vi "prepDO_focusalign.vi"(2 "rate":dbl=30000.0 format="%#_13g", 3 "data":digitalwaveform[](array[waveform]), 4 "bufferAO":i32) -> (0 "error out":errorcluster, 1 "task out":refnum<k21>)   [LabVIEW 2015]
uses:
  <vilib>/DAQmx/write.llb/DAQmx Write (Digital 1D Wfm NChan NSamp).vi
  <vilib>/DAQmx/create/channels.llb/DAQmx Create Channel (DO-Digital Output).vi
  <vilib>/DAQmx/configure/timing.llb/DAQmx Timing (Sample Clock).vi
  <vilib>/Waveform/DWDTOps.llb/DWDT Uncompress Digital.vi
  <vilib>/DAQmx/miscellaneous.llb/DAQmx Fill In Error Info.vi
panel:
  in  "error in":errorcluster
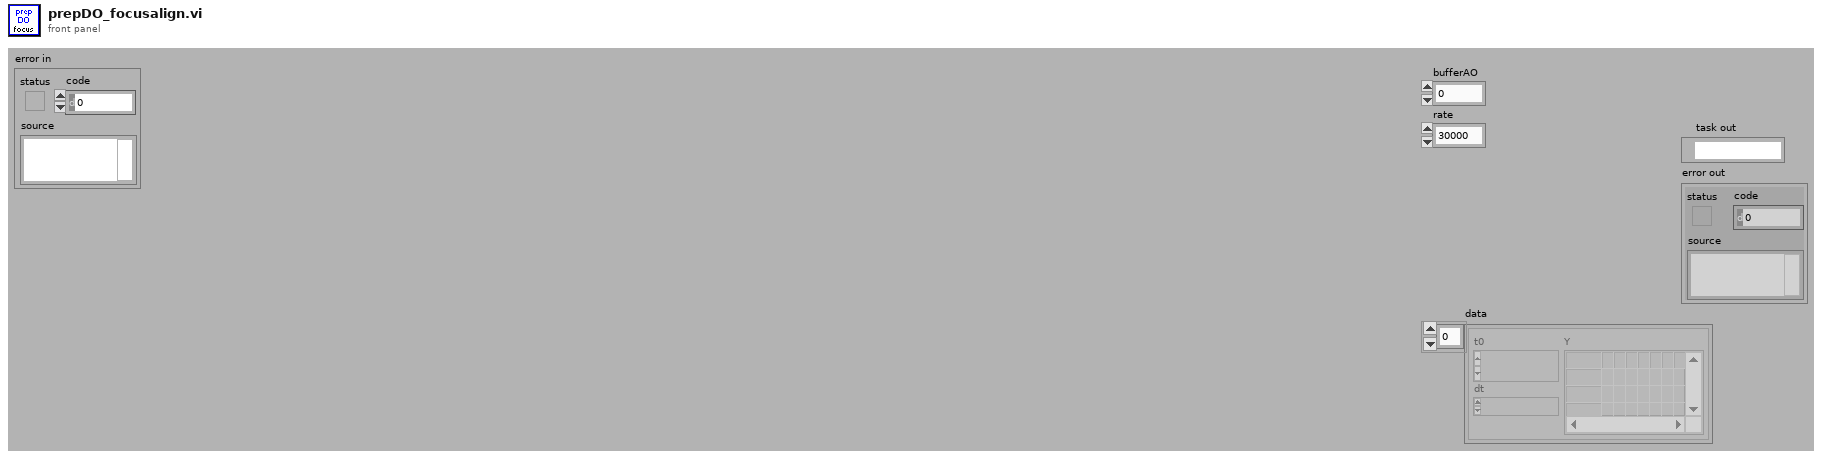
[diagram p1: front panel]
types:
  T1 = cluster{"StageS":i32, "StageL":i32, "currmeas data dir":path, "image OD":u16, "contour OD":u16, "point OD":u16, "AOlines":tag[], "AIlines":tag[], "CI lines":tag[], "DO lines":tag[], "AO names":string[], "CI names":string[], "AI names":string[], "DO names":string[], "CIextensions":string[], "AIextensions":string[], "Voltage to Ygalvo":i32, "Voltage to Xgalvo":i32, "Voltage to patch":i32, "640 shutter":i32, "2P shutter":i32, "LT timestamp":u32, "Vp":i32, "Ip":i32, "camera trigger":i32, "master data dir":path, "voltage to Zpos":i32, "Vto2P":i32, "640 AO":i32, "488 AO":i32, "532 AO":i32, "640TTL":u32, "488TTL":u32, "532TTL":u32, "Device 1 sampleclock out":tag, "Device 1 Starttrigger out":tag, "Device 2 sampleclock in":tag, "Device 2 StartTrigger in ":tag, "2PODTTL":u32, "488 shutter":u32, "LCVR red":u32, "LCVR blue":u32}
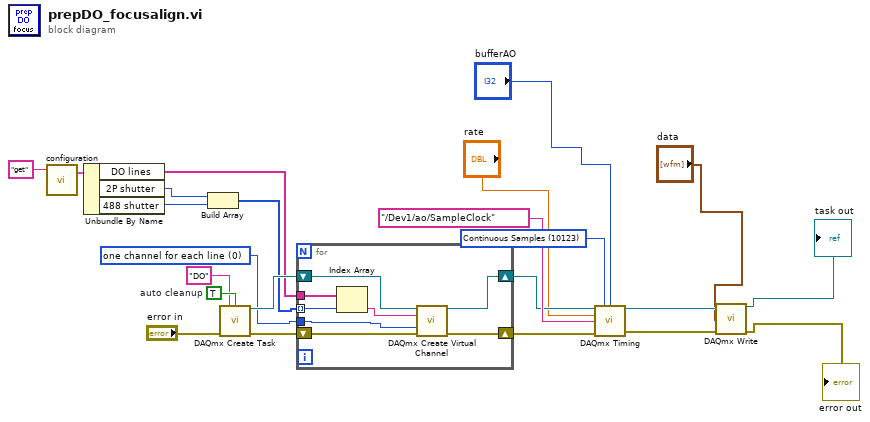
[diagram p0: block diagram]
diagram:
  w7 = 10123 items=["Finite Samples"=10178, "Continuous Samples"=10123, "Hardware Timed Single Point"=12522] ("sample mode")
  w13 = 0 items=["one channel for each line", "one channel for all lines"] ("line grouping")
  w22 = TRUE  # auto cleanup
  n1 = call "configuration.vi"("command"="get") -> ("config out"=w15:T1)  [unwired: 2 in, 1 out]
  n2 = Unbundle By Name(w15) -> ("DO lines"=w14:tag[], "2P shutter"=w5:i32, "488 shutter"=w4:u32)
  n3 = Build Array(w5, w4) -> (w3:u32[])
  n4 = call <vilib>:"DAQmx Create Task.vi"("new task name"="DO", "auto cleanup"=w22, "error in"="error in") -> ("task out"=w23:refnum<k21>, "error out"=w21:errorcluster)  [unwired: 11 in]
  n5 = for {
    shift-right: [w26] -> w17
    shift-left: w21 -> [w30]
    tunnel: w3 -> [w29] mode=indexing
    shift-right: [w27] -> w18
    shift-left: w23 -> [w31]
    tunnel: w14 -> [w25]
    tunnel: w13 -> [w24]
    n6 = Index Array(array=w25, index=w29) -> (element=w28:tag)
    n7 = call-poly <vilib>:"DAQmx Create Virtual Channel.vi"("task in"=w31, "lines"=w28, "line grouping"=w24, "error in"=w30) -> ("task out"=w27:refnum<k21>, "error out"=w26:errorcluster)  [unwired: 10 in]
  }
  n8 = call-poly <vilib>:"DAQmx Timing.vi"("task/channels in"=w18, "sample mode"=w7, "samples per channel"="bufferAO", "rate"="rate", "source"=tag "/Dev1/ao/SampleClock", "error in"=w17) -> ("task out"=w12:refnum<k21>, "error out"=w11:errorcluster)  [unwired: 1 in, 7 out]
  n9 = call-poly <vilib>:"DAQmx Write.vi"("task/channels in"=w12, "data"="data", "error in"=w11) -> ("task out"=→"task out":refnum<k21>, "error out"=→"error out":errorcluster)  [unwired: 10 in, 1 out]
